vi "Mark Special Table Cell.vi"(7 "Normal":u32(colorbox)=16448250, 8 "error in (no error)":errorcluster caption="错误输入（无错误）", 9 "Mark":u32(colorbox)=16711680, 10 "Mark Array":bool[][](array[boolean]), 11 "Table Ref In":refnum<vi>) -> (0 "error out":errorcluster caption="错误输出", 3 "Table Ref Out":refnum<vi>)   [LabVIEW 2013, in "Table Tool.lvlib"]
uses:
  Table Tool.lvlib
  Custum Type/GetOrSet.ctl
  Property/Set Or get ActiveCell Bk Color.vi
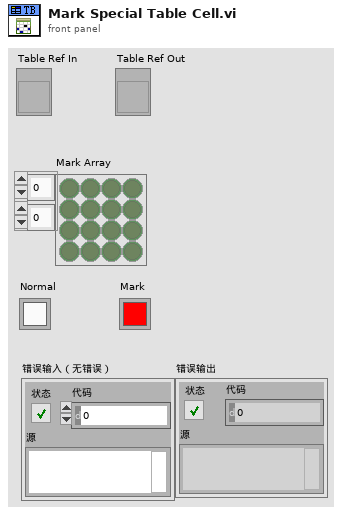
[diagram p1: front panel]
types:
  T1 = typedef "Table Tool.lvlib/GetOrSet.ctl" = enum16{"Get", "Set"}
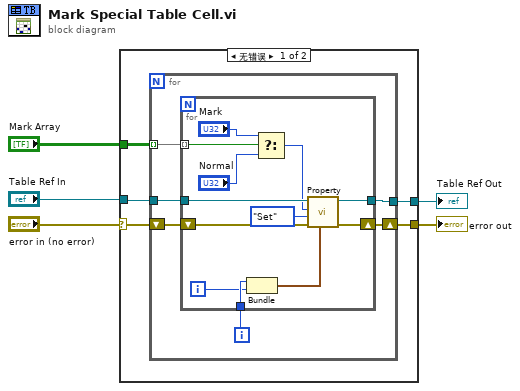
[diagram p0: block diagram]
diagram:
  n1 = case shown="无错误" "error in (no error)" {
    selector: "error in (no error)" -> [w8 w30]
    tunnel: "Table Ref In" -> [w9 w29]
    tunnel: [w6 w29] -> w3
    tunnel: [w7 w30] -> w2
    tunnel: "Mark Array" -> [w10 _]
    frame No Error {
      n2 = for {
        tunnel: w10 -> [w16] mode=indexing
        tunnel: w9 -> [w15]
        shift-right: [w13] -> w7
        shift-left: w8 -> [w14]
        tunnel: [w12] -> w6
        i -> [w11]
        n3 = for {
          tunnel: w16 -> [w24] mode=indexing
          tunnel: w15 -> [w28]
          shift-right: [w26] -> w13
          shift-left: w14 -> [w27]
          tunnel: [w25] -> w12
          tunnel: w11 -> [w19]
          i -> [w18]
          n4 = Bundle(w19, w18) -> (w17:cluster{i32, i32})  [unwired: 1 in]
          n5 = Select(t="Mark", s=w24, f="Normal") -> (s? t:f=w21:u32)
          n6 = call-poly "Property.vi"("Active Cell"=w17, "error in (no error)"=w27, "Mode"=GetOrSet."Set", "BK Color In"=w21, "Table Ref In"=w28) -> ("error out"=w26:errorcluster, "Table Ref Out"=w25:refnum<vi>)  [unwired: 4 in, 1 out]
        }
      }
    }
    frame Error {
    }
  }
  "Table Ref Out" <- w3
  "error out" <- w2
